vi "New Console Session.vi"(6 "Persist After Shutdown?(F)":bool, 7 "Format Specifier":string="%T[TIME] - %s[LVL] - %s[ID] - %s[EVT] ", 8 "error in (no error)":errorcluster, 11 "UI Config":T1={"BG Color"=16448250, "Text Color"=3421236, "Font Size"=18, "Bold?"=TRUE}) -> (0 "error out":errorcluster, 2 "ConsoleSink out":refnum<class "ConsoleSink.lvclass">, 3 "ConsoleSession out":refnum<class "ConsoleSession.lvclass">)   [LabVIEW 2017, in "ConsoleView.lvlib" / "ConsoleSession.lvclass"]
doc: "Create a new console session. Inject the console sink into a log instance to get a live stream view of log events with dynamic filtering capabilities. The session class can be used to dynamically show or hide the view, and to close the view and sink. If these features are not used, maintaining the session class in caller code is not required - the view and all associated references will be closed with the log instance, assuming the Persist After Shutdown flag is false.\n\nIf the Persist After Shutdown flag is true, the console view will remain open after the logger is stopped until explicitly closed by the user."
uses:
  <vilib>/gpm_packages/@cs/event-logger/Source/ConsoleView/ConsoleInterface/ConsoleSession.lvclass
  <vilib>/gpm_packages/@cs/event-logger/Source/ConsoleView/Sink/ConsoleSink.lvclass
  <vilib>/gpm_packages/@cs/event-logger/Source/ConsoleView/View/TypeDef/String Config.ctl
  <vilib>/gpm_packages/@cs/event-logger/Source/Composed Log/Log Sink/Sink Error Actions ENUM.ctl
  <vilib>/gpm_packages/@cs/event-logger/Source/Composed Log/Types/Log Level.ctl
  <vilib>/gpm_packages/@cs/event-logger/Source/Composed Log/Types/MessageCluster.ctl
  <vilib>/gpm_packages/@cs/event-logger/Source/String Formats/String Expression Format/String Expression Format.lvclass/String Expression Format.ctl
  <vilib>/gpm_packages/@cs/event-logger/Source/ConsoleView/ConsoleInterface/ConsoleSession.lvclass/ConsoleSession.ctl
  <vilib>/gpm_packages/@cs/event-logger/Source/String Formats/String Expression Format/Run Formatter.vi
  <vilib>/dlg_ctls.llb/Space Constant.vi
  <vilib>/gpm_packages/@cs/event-logger/Source/String Formats/String Expression Format/String Expression Format.lvclass
  C:/Program Files/National Instruments/LabVIEW 2017/vi.lib/gpm_packages/@cs/event-logger/Source/IStringFormat/IStringFormat.lvclass
  <vilib>/gpm_packages/@cs/event-logger/Source/ConsoleView/View/ConsoleView.lvclass
  <vilib>/gpm_packages/@cs/event-logger/Source/Composed Log/Log Sink/Log Sink.lvclass
  <vilib>/gpm_packages/@cs/event-logger/Source/Composed Log/Composed Log.lvlib
panel:
  # "Use me to dynamically show/hide the view."
  # "Inject me into the logger"
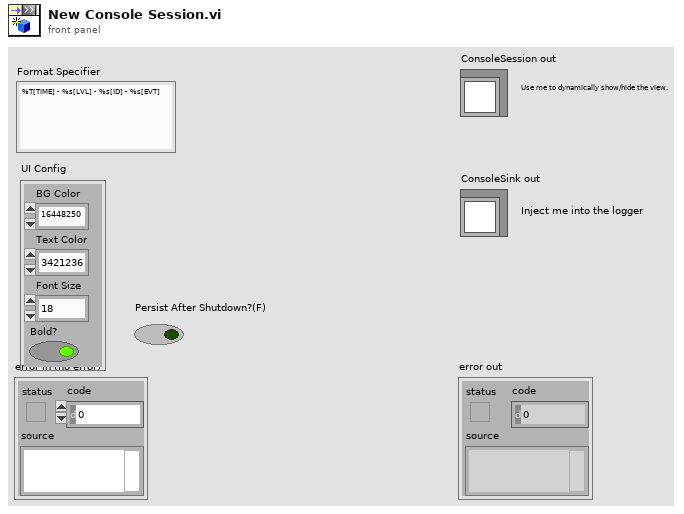
[diagram p1: front panel]
types:
  T1 = typedef "ConsoleView.lvlib/ConsoleView.lvclass/String Config.ctl" = cluster{"BG Color":u32, "Text Color":u32, "Font Size":u32, "Bold?":bool}
  T2 = typedef "Composed Log.lvlib/MessageCluster.ctl" = cluster{"Message":string, "Data":variant}
  T3 = typedef "Composed Log.lvlib/Log Level.ctl" = enum16{"Debug", "Info", "Warning", "Error", "Critical"}
  T4 = typedef "Composed Log.lvlib/Log Sink.lvclass/Sink Error Actions ENUM.ctl" = enum16{"Ignore Error and Continue", "Ignore Error and Close Sink", "Report Error and Close Sink"}
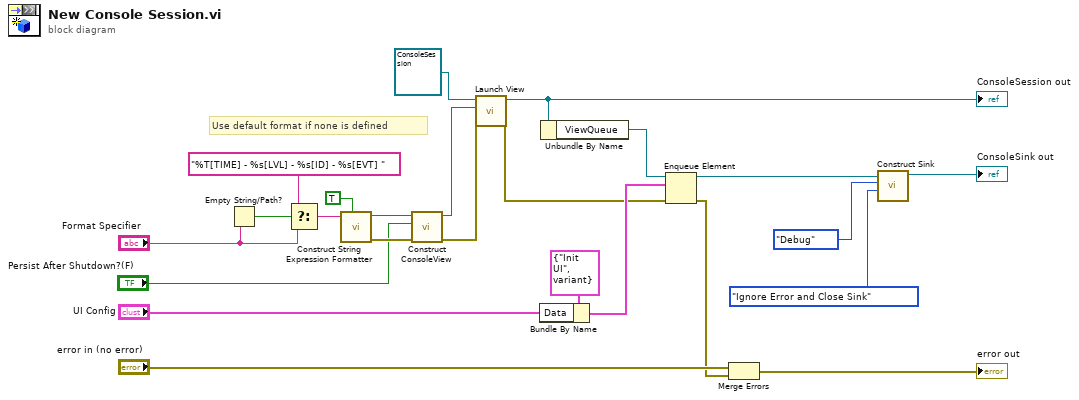
[diagram p0: block diagram]
diagram:
  # "Use default format if none is defined"
  n1 = Empty String/Path?(string/path="Format Specifier") -> (empty?=w5:bool)
  n2 = Select(t="%T[TIME] - %s[LVL] - %s[ID] - %s[EVT] " ("Format Specifier"), s=w5, f="Format Specifier") -> (s? t:f=w2:string)
  n3 = call <vilib>:"Construct String Expression Formatter.vi"("Append EOL?"=TRUE, "Format Specifier"=w2) -> ("error out"=w14:errorcluster, "String Expression Format out"=w15:refnum<class "String Expression Format.lvclass">)  [unwired: 8 in]
  n4 = call <vilib>:"Construct ConsoleView.vi"("error in (no error)"=w14, "Persist after shutdown?"="Persist After Shutdown?(F)", "StringFormat"=w15) -> ("error out"=w13:errorcluster, "ConsoleView out"=w22:refnum<class "ConsoleView.lvclass">)  [unwired: 7 in]
  n5 = call <vilib>:"Launch View.vi"("error in (no error)"=w13, "ConsoleView in"=w22, "ConsoleInterface in"=refnum<class "ConsoleSession.lvclass"> refnum) -> ("error out"=w8:errorcluster, "ConsoleInterface out"=w21:refnum<class "ConsoleSession.lvclass">)  [unwired: 7 in]
  "ConsoleSession out" <- w21
  n6 = Bundle By Name(cluster=T2 {"Message"="Init UI", "Data"=variant} ("element"), "Data"="UI Config") -> (w10:T2)
  n7 = Unbundle By Name(w21) -> ("ViewQueue"=w20:refnum<queue>)
  n8 = Enqueue Element(queue=w20, element=w10, error in (no error)=w8) -> (queue out=w12:refnum<queue>, error out=w6:errorcluster)  [unwired: 1 in, 1 out]
  n9 = Merge Errors("error in (no error)", w6) -> (→"error out":errorcluster)
  n10 = call <vilib>:"Construct Sink.vi"("Error Action"=Sink_Error_Actions_ENUM."Ignore Error and Close Sink", "LogLevel"=Log_Level."Debug", "ViewQueue"=w12) -> ("ConsoleSink out"=→"ConsoleSink out":refnum<class "ConsoleSink.lvclass">)  [unwired: 8 in]
